vi "Write SubVI Reference.vi"(8 "error in (no error)":errorcluster, 10 "SubVI Reference":refnum<vi>, 11 "SubVIConverter in":refnum<class "SubVIConverter.lvclass">) -> (0 "error out":errorcluster, 3 "SubVIConverter out":refnum<class "SubVIConverter.lvclass">)   [LabVIEW 2017, in "SubVIConverter.lvclass"]
uses:
  SubVIConverter.lvclass
  SubVIConverter.lvclass/SubVIConverter.ctl
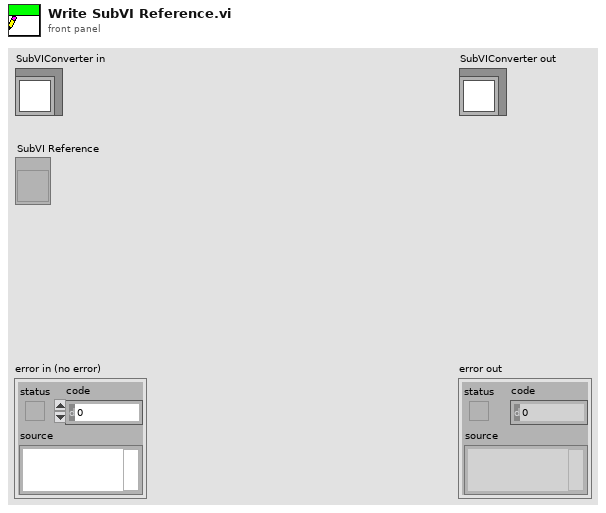
[diagram p1: front panel]
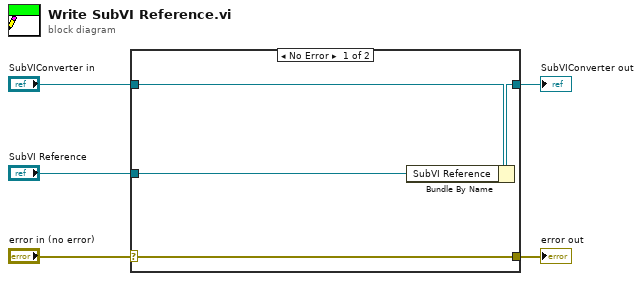
[diagram p0: block diagram]
diagram:
  n1 = case shown="No Error" "error in (no error)" {
    selector: "error in (no error)" -> [w9 w10]
    tunnel: [w9 w10] -> w4
    tunnel: [w7 w11] -> w2
    tunnel: "SubVIConverter in" -> [w8 w11]
    tunnel: "SubVI Reference" -> [w6 _]
    frame No Error {
      n2 = Bundle By Name(cluster=w8, "SubVI Reference"=w6) -> (w7:refnum<class "SubVIConverter.lvclass">)
    }
    frame Error {
    }
  }
  "error out" <- w4
  "SubVIConverter out" <- w2
